vi "FormatToJSON.vi"(8 "Error In":errorcluster, 9 "Post_command":string, 11 "Sid":dbl) -> (0 "Error Out":errorcluster, 2 "POST_command_sid_only":string, 3 "Final_POST_Command":string)   [LabVIEW 2017]
doc: "<B>Sid:</B>\n Session id generated at runtime by webserver and LabVIEW will fetch Sid from webserver and store this it in UltraSonic_Global_Config.ini. \n Path: \\UltraSonic_Test_Scripts\\UltraSonic_Global_Config.ini\n\n<B>Post_command :</B> \nPOST_command is to fetch values from the web server like system info, version, weld recipe parameters etc.,\nPOST_command should be as per the requirement in JSON format except session ID\n\nFor example: {\"parameter1\":value1,\"parameter2\":value2,...}\n\nThe session id will be concatinated by LabVIEW during runtime, user need not worry of the session id\n\n<B>Final_POST_Command : </B>\nThis string output is concatenation of Sid and Post_command and it will be formated to JSON format, suitable to communicate to webserver.\n\nFor example: {\"Sid\":12345,\"ParamId\":177,\"ParamValue\":0.250,\"Reason\":\"xyz\"}"
panel:
  # "Concatenate Sid [session ID] and post command from \nini file  and format it into JSON format suitable to send to webserver:"
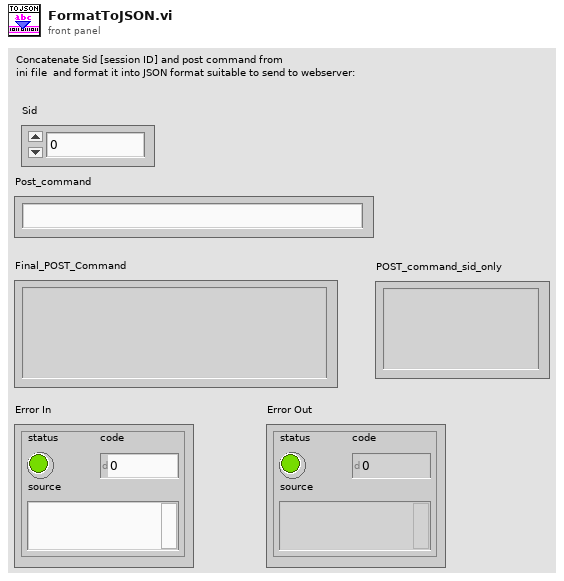
[diagram p1: front panel]
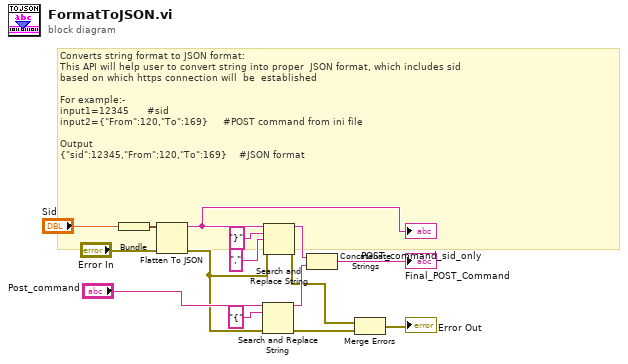
[diagram p0: block diagram]
diagram:
  # "Converts string format to JSON format:\nThis API will help user to convert string into proper  JSON format, which includes sid \nbased on which https connection will  be  established\n\nFor example:-\ninput1=12345      #sid\ninput2={\"From\":120,\"To\":169}     #POST command from ini file\n\nOutput\n{\"sid\":12345,\"From\":120,\"To\":169}    #JSON format"
  n1 = Bundle("Sid"="Sid") -> (w15:cluster{"Sid":dbl})  [unwired: 1 in]
  n2 = Flatten To JSON(anything=w15, error in (no error)="Error In") -> (JSON string=w1:string, 11:w5:errorcluster)  [unwired: 1 in]
  "POST_command_sid_only" <- w1
  n3 = Search and Replace String(input string="Post_command", search string="{", error in=w5) -> (result string=w10:string, error out=w3:errorcluster)  [unwired: 5 in, 2 out]
  n4 = Search and Replace String(input string=w1, search string="}", replace string="," ("replace string (\"\")"), error in=w5) -> (result string=w9:string, error out=w4:errorcluster)  [unwired: 4 in, 2 out]
  n5 = Concatenate Strings(w9, w10) -> (→"Final_POST_Command":string)
  n6 = Merge Errors(w4, w3) -> (→"Error Out":errorcluster)
